vi "ReadBankNode.vi"(8 "Error In":errorcluster, 11 "Bank Node In":refnum<k20>) -> (0 "Error Out":errorcluster, 2 "Bank Configuration":T1, 3 "Bank Node Out":refnum<k20>)   [LabVIEW 2012]
uses:
  BankConfiguration.ctl
  <vilib>/xml/NI_XML.lvlib
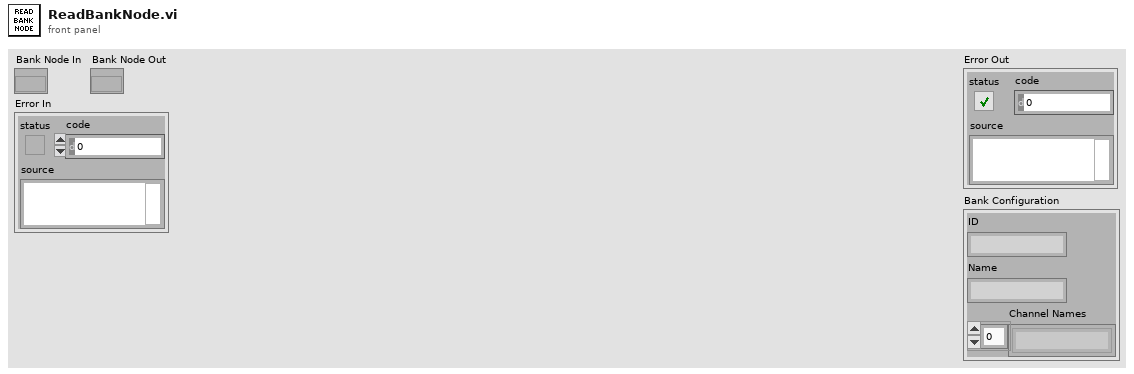
[diagram p1: front panel]
types:
  T1 = typedef "BankConfiguration.ctl" = cluster{"ID":string, "Name":string, "Channel Names":string[]}
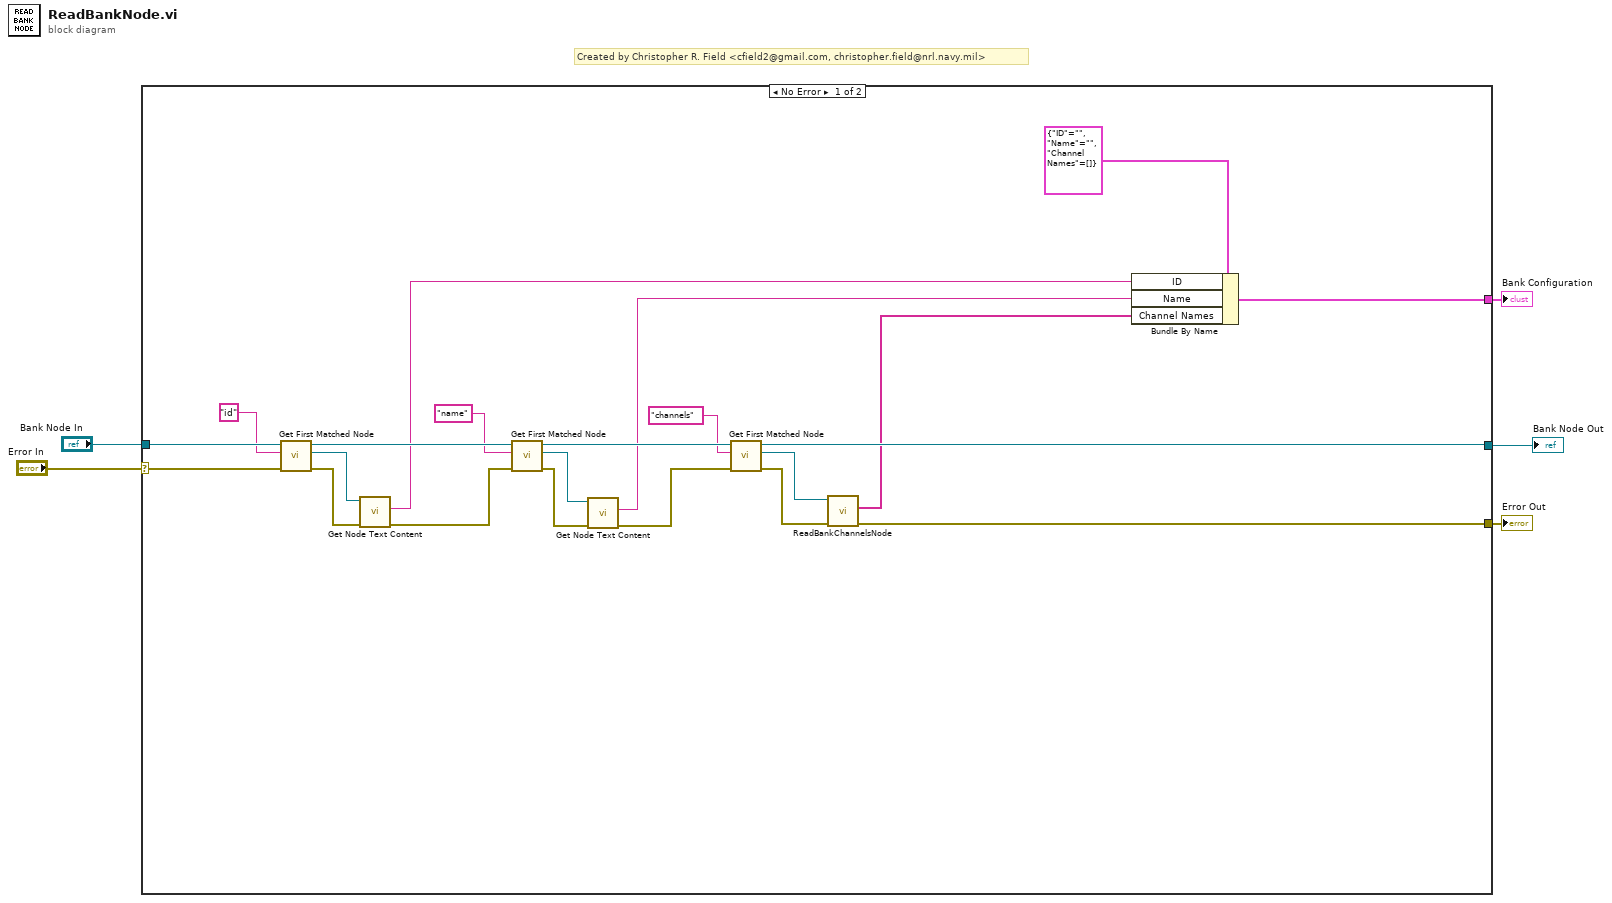
[diagram p0: block diagram]
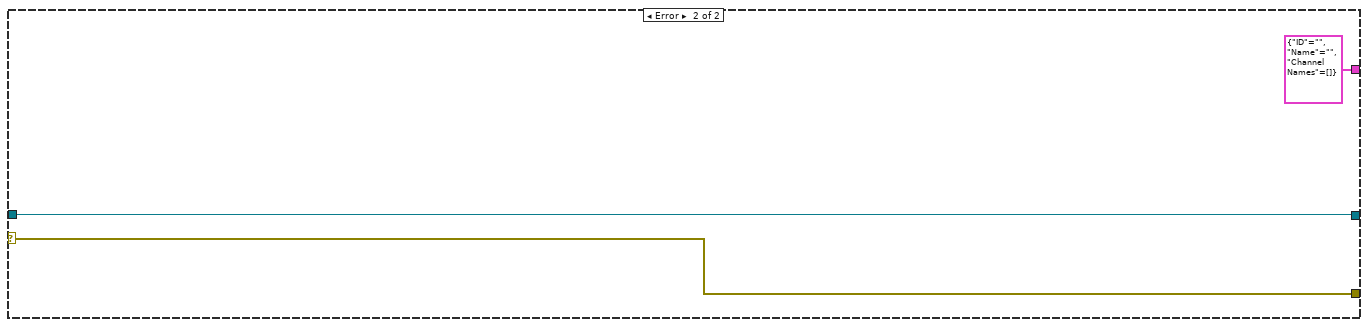
[diagram p2: hidden frame]
diagram:
  # "Created by Christopher R. Field <cfield2@gmail.com, christopher.field@nrl.navy.mil>"
  n1 = case shown="No Error" "Error In" {
    selector: "Error In" -> [w25 w29]
    tunnel: "Bank Node In" -> [w27 w30]
    tunnel: [w12 w30] -> w3
    tunnel: [w11 w29] -> w2
    tunnel: [w6 T1 {"ID"="", "Name"="", "Channel Names"=[]} ("Bank Configuration")] -> w1
    frame No Error {
      n2 = call <vilib>:"Get First Matched Node.vi"("error in (no error)"=w25, "XPath expression"="id", "node in"=w27) -> ("error out"=w23:errorcluster, "node result"=w24:refnum<k20>, "node out"=w21:refnum<k20>)  [unwired: 6 in]
      n3 = call <vilib>:"Get Node Text Content.vi"("error in (no error)"=w23, "node in"=w24) -> ("error out"=w22:errorcluster, "node text"=w9:string)  [unwired: 7 in, 1 out]
      n4 = call <vilib>:"Get First Matched Node.vi"("error in (no error)"=w22, "XPath expression"="name", "node in"=w21) -> ("error out"=w18:errorcluster, "node result"=w19:refnum<k20>, "node out"=w17:refnum<k20>)  [unwired: 6 in]
      n5 = call <vilib>:"Get Node Text Content.vi"("error in (no error)"=w18, "node in"=w19) -> ("error out"=w15:errorcluster, "node text"=w8:string)  [unwired: 7 in, 1 out]
      n6 = call <vilib>:"Get First Matched Node.vi"("error in (no error)"=w15, "XPath expression"="channels", "node in"=w17) -> ("error out"=w13:errorcluster, "node result"=w14:refnum<k20>, "node out"=w12:refnum<k20>)  [unwired: 6 in]
      n7 = call "ReadBankChannelsNode.vi"("Error In"=w13, "Channels Node In"=w14) -> ("Error Out"=w11:errorcluster, "Channel Names"=w7:string[])  [unwired: 7 in, 1 out]
      n8 = Bundle By Name(cluster=T1 {"ID"="", "Name"="", "Channel Names"=[]} ("Bank Configuration"), "ID"=w9, "Name"=w8, "Channel Names"=w7) -> (w6:T1)
    }
    frame Error {
    }
  }
  "Bank Node Out" <- w3
  "Error Out" <- w2
  "Bank Configuration" <- w1
